vi "BLE_Thread.vi"(9 "ble queue in":refnum<queue>, 11 "controller queue out":refnum<queue>) -> ()   [LabVIEW 2020]
uses:
  BLE_Request.ctl
  BLE_Request_Command.ctl
  Controller_Request.ctl
  Controller_Request_Command.ctl
  BLE_Action.ctl
  BLE_Data_Packet.ctl
  BLE_Data.ctl
  C:/Users/Trait/Repos/BLE_BeaconSensor/BLE_ClientPC/BLELib.dll
  BLELib.dll
  BLE.lvlib
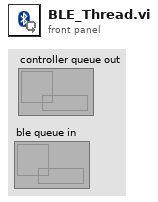
[diagram p1: front panel]
types:
  T1 = typedef "Controller_Request.ctl" = cluster{"Command":T2, "Parameter":variant}
  T2 = typedef "Controller_Request_Command.ctl" = enum16{"BLE_ScannedDevices", "BLE_ConnectionResult", "BLE_NotificationToogleResult", "BLE_NotificationData", "BLE_ConnTimeout", "BLE_CloseResult", "User_Init", "User_ScanRequest", "User_ConnectionRequest", "User_CloseRequest", "User_NotficationToggleRequest"}
  T3 = typedef "BLE_Action.ctl" = enum16{"Idle", "Notify", "Scan"}
  T4 = typedef "BLE_Data.ctl" = cluster{".NET Ref":refnum<k24>, "BLE action":T3, "Timeout":u32, "UUIDs":cluster{"TEMP":string, "ACC X":string, "ACC Y":string, "ACC Z":string}}
  T5 = typedef "BLE_Request.ctl" = cluster{"Command":T6, "Parameter":variant}
  T6 = typedef "BLE_Request_Command.ctl" = enum16{"BLE_Idle", "BLE_Init", "BLE_ScanToogle", "BLE_Connect", "BLE_NotificationToogle", "BLE_Close"}
  T7 = cluster{"TEMP":string, "ACC X":string, "ACC Y":string, "ACC Z":string}
  T8 = typedef "BLE_Data_Packet.ctl" = cluster{"Temperature":cluster{"Available":bool, "Value":sgl}, "Acceleration X":cluster{"Available":bool, "Value":i16}, "Acceleration Y":cluster{"Available":bool, "Value":i16}, "Acceleration Z":cluster{"Available":bool, "Value":i16}}
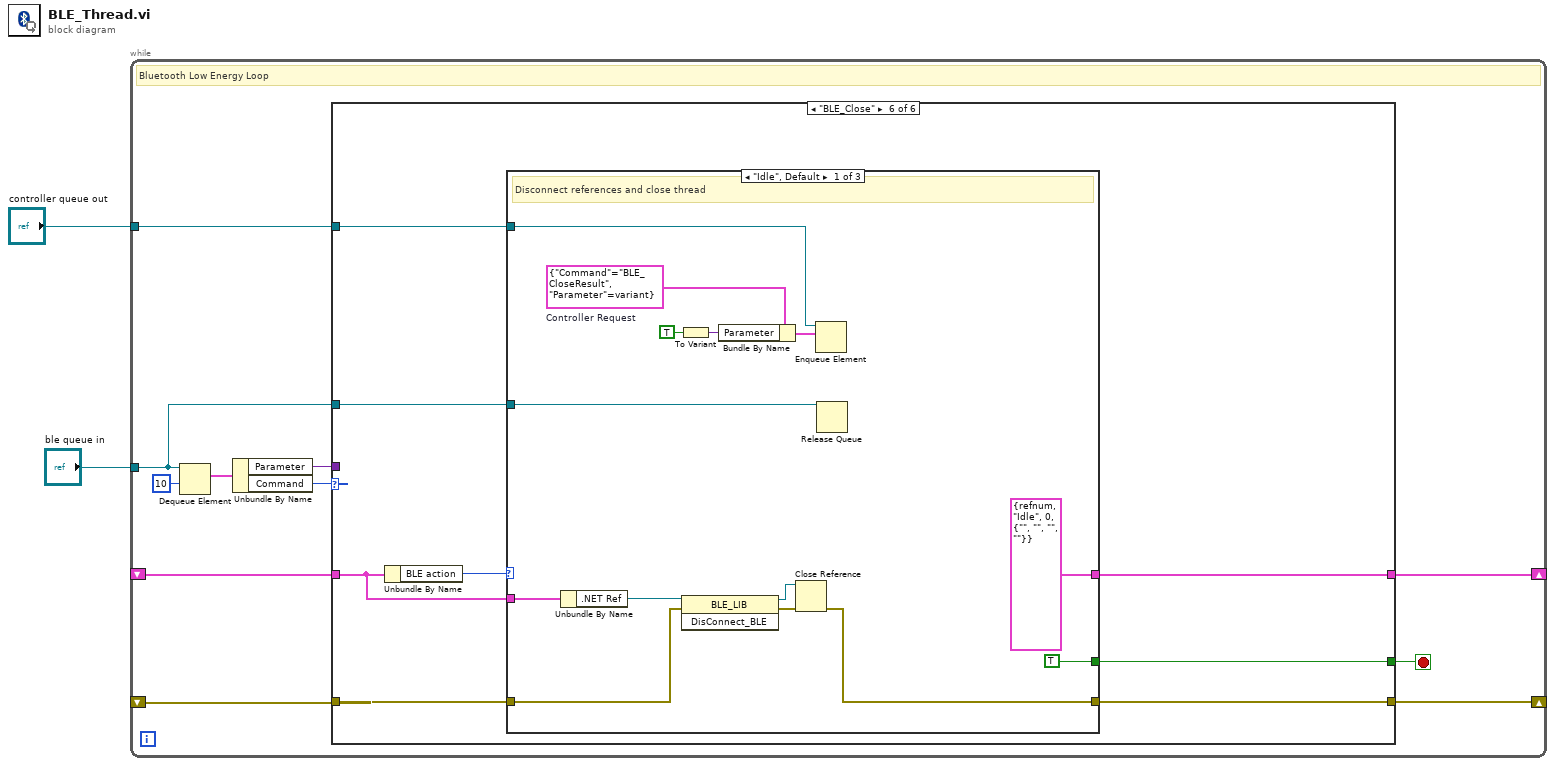
[diagram p0: block diagram]
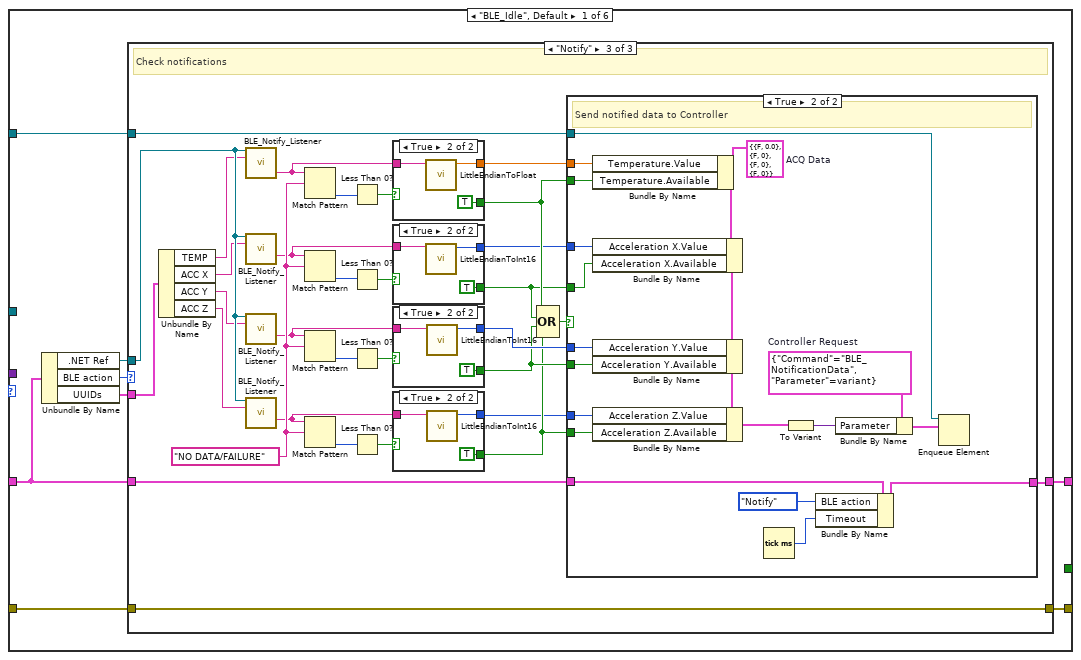
[diagram p2: hidden frame]
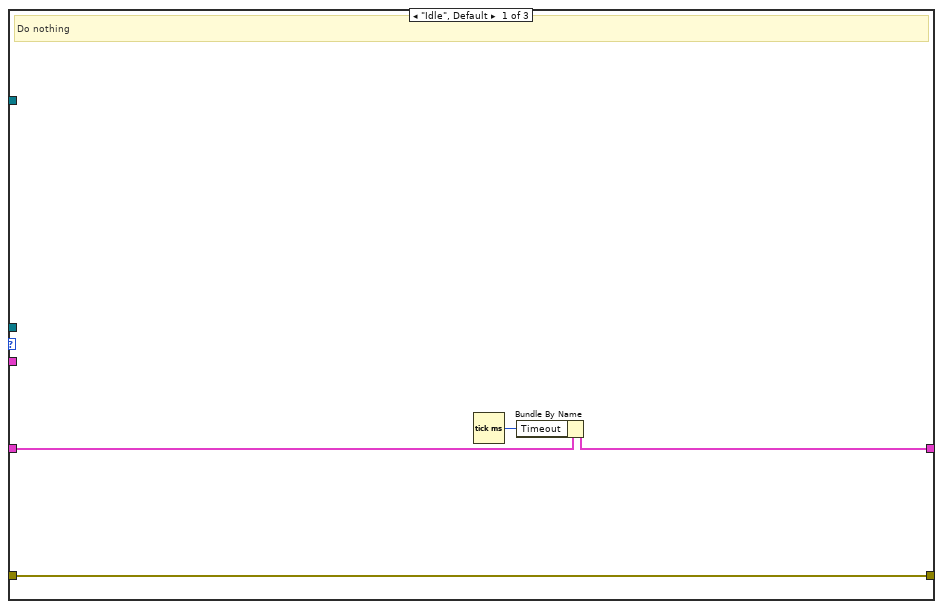
[diagram p3: hidden frame]
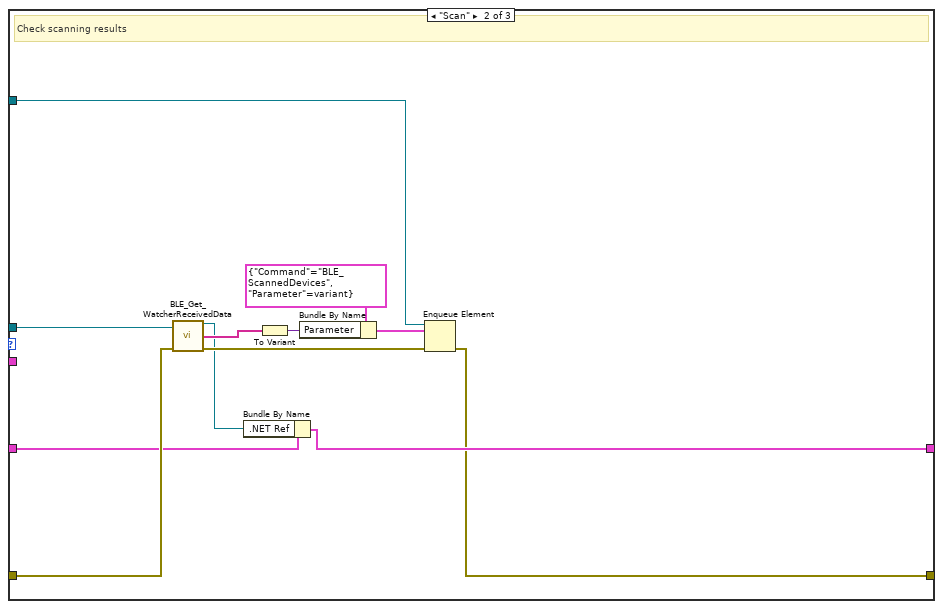
[diagram p4: hidden frame]
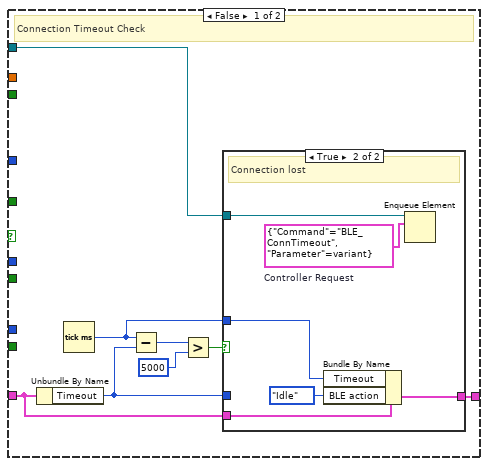
[diagram p5: hidden frame]
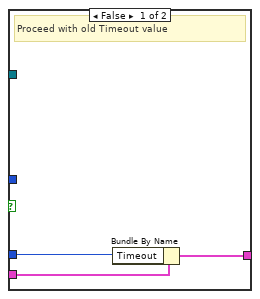
[diagram p6: hidden frame]
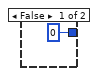
[diagram p7: hidden frame]
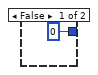
[diagram p8: hidden frame]
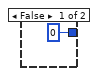
[diagram p9: hidden frame]
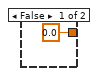
[diagram p10: hidden frame]
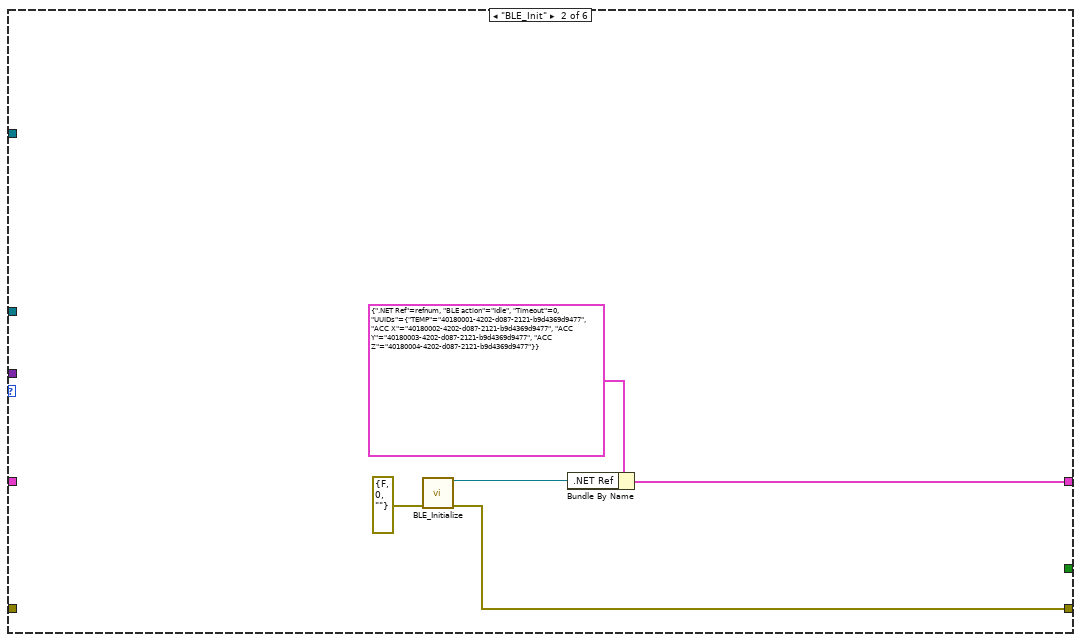
[diagram p11: hidden frame]
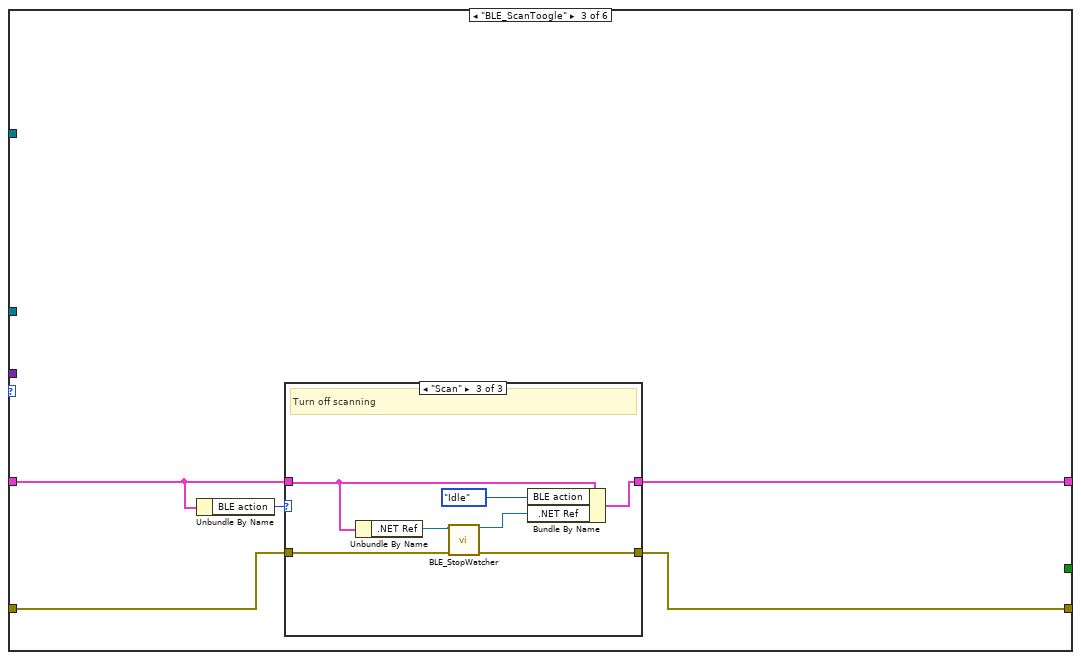
[diagram p12: hidden frame]
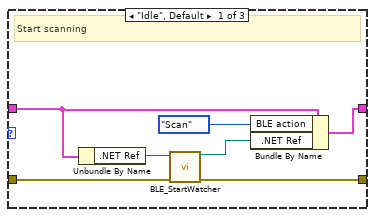
[diagram p13: hidden frame]
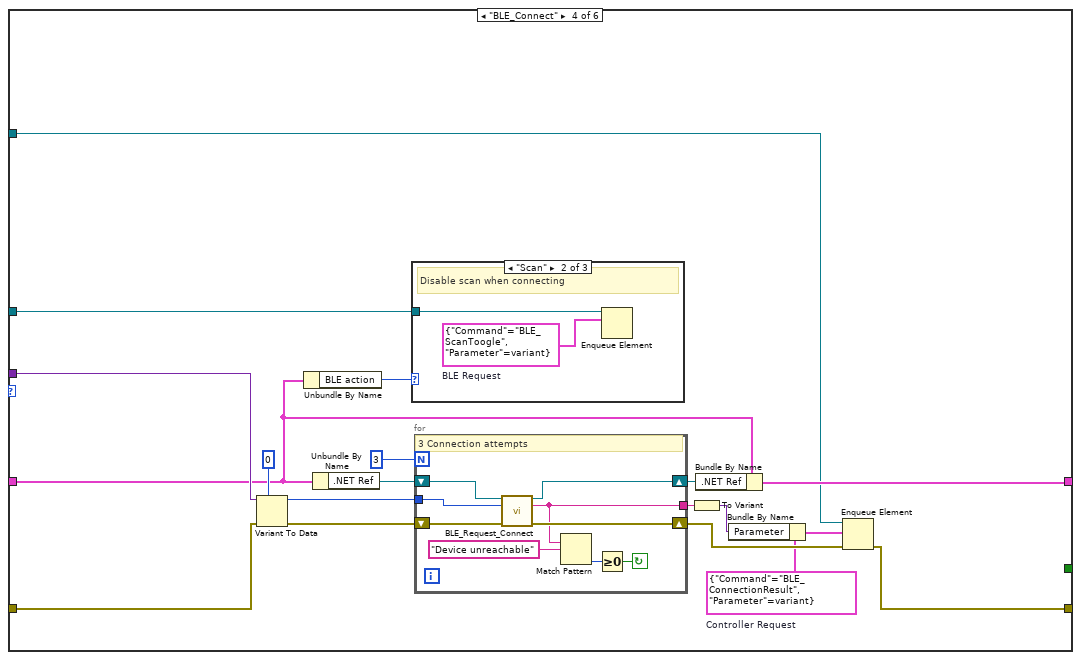
[diagram p15: hidden frame]
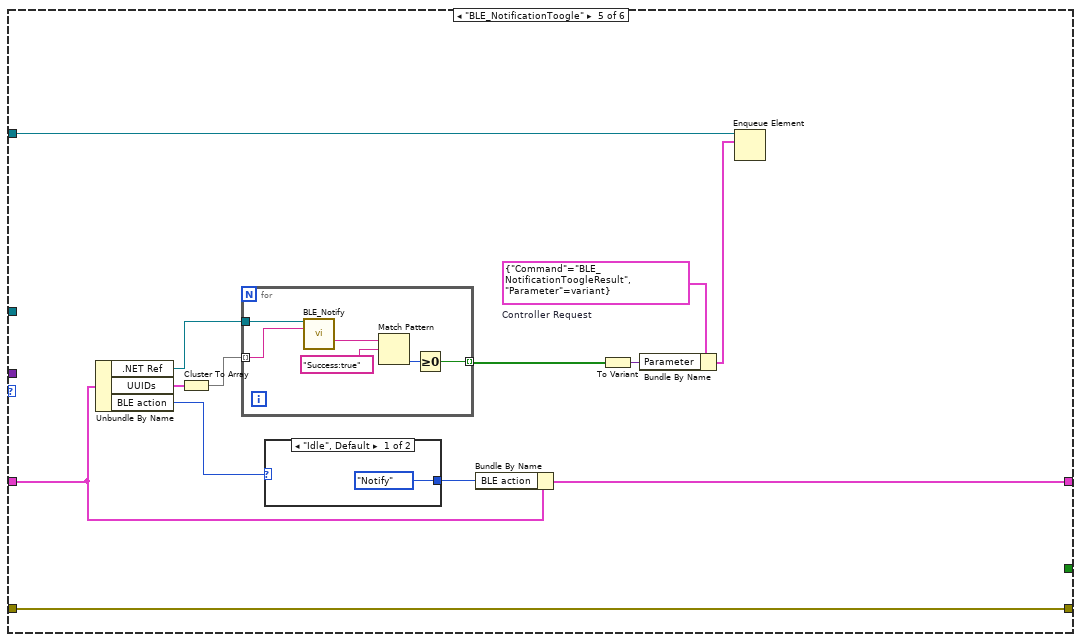
[diagram p18: hidden frame]
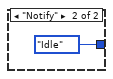
[diagram p19: hidden frame]
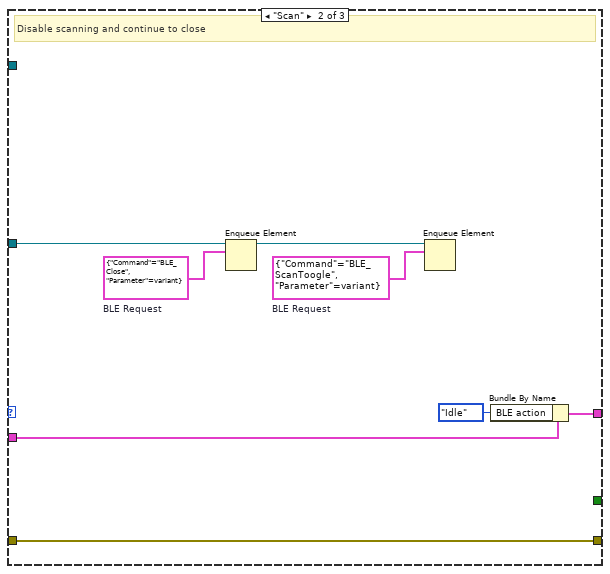
[diagram p20: hidden frame]
diagram:
  n1 = while {
    shift-right: [w4] -> _
    shift-left: _ -> [w8]
    shift-right: [w13] -> _
    shift-left: _ -> [w12]
    tunnel: "ble queue in" -> [w6]
    tunnel: "controller queue out" -> [w3]
    stop <- w5 stop-if-true
    # "Bluetooth Low Energy Loop"
    n2 = Dequeue Element(queue=w6, timeout in ms (-1)=10) -> (element=w10:T5)  [unwired: 1 in, 3 out]
    n3 = Unbundle By Name(w10) -> ("Parameter"=w7:variant, "Command"=w9:T6)
    n4 = case shown="\"BLE_Close\"" w9 {
      tunnel: w12 -> [w20 _ w130 w164 w192 w204]
      tunnel: [w16 w128 w129 w153 w192 w203] -> w13
      tunnel: [w17 w126 w133 w160 w190 w206] -> w4
      tunnel: w8 -> [w15 _ w132 w157 w191 w205]
      tunnel: w7 -> [_ _ _ w167 _ _]
      tunnel: w6 -> [_ _ _ w155 _ w207]
      tunnel: [_ _ _ _ _ w202] -> w5
      tunnel: w3 -> [w18 _ _ w152 w189 w201]
      frame "BLE_Idle", Default {
        n5 = Unbundle By Name(w15) -> (".NET Ref"=w19:refnum<k24>, "BLE action"=w21:T3, "UUIDs"=w14:T7)
        n6 = case shown="\"Notify\"" w21 {
          tunnel: w20 -> [w25 w37 w69]
          tunnel: [w25 w31 w69] -> w16
          tunnel: w15 -> [w24 w27 w39]
          tunnel: [w23 w35 w38] -> w17
          tunnel: w19 -> [_ w28 w67]
          tunnel: w18 -> [_ w29 w40]
          tunnel: w14 -> [_ _ w68]
          frame "Idle", Default {
            # "Do nothing"
            n7 = Tick Count (ms)() -> (millisecond timer value=w22:u32)
            n8 = Bundle By Name(cluster=w24, "Timeout"=w22) -> (w23:T4)
          }
          frame "Scan" {
            # "Check scanning results"
            n9 = call "BLE_Get_WatcherReceivedData.vi"(".NET Refnum in"=w28, "error in (no error)"=w37) -> (".NET Refnum out"=w26:refnum<k24>, "Bluetooth Addr"=w33:string[], "error out"=w32:errorcluster)  [unwired: 6 in, 5 out]
            n10 = Bundle By Name(cluster=w27, ".NET Ref"=w26) -> (w35:T4)
            n11 = To Variant(anything=w33) -> (Variant=w36:variant)
            n12 = Bundle By Name(cluster=T1 {"Command"=enum."BLE_ScannedDevices", "Parameter"=variant}, "Parameter"=w36) -> (w30:T1)
            n13 = Enqueue Element(queue=w29, element=w30, error in (no error)=w32) -> (error out=w31:errorcluster)  [unwired: 1 in, 2 out]
          }
          frame "Notify" {
            w55 = "NO DATA/FAILURE" ("regular expression")
            # "Check notifications"
            n14 = Unbundle By Name(w68) -> ("TEMP"=w66:string, "ACC X"=w65:string, "ACC Y"=w64:string, "ACC Z"=w63:string)
            n15 = call "BLE_Notify_Listener.vi"(".NET Refnum in"=w67, "UUID"=w66) -> ("Result"=w52:string)  [unwired: 11 in, 2 out]
            n16 = call "BLE_Notify_Listener.vi"(".NET Refnum in"=w67, "UUID"=w65) -> ("Result"=w53:string)  [unwired: 11 in, 2 out]
            n17 = call "BLE_Notify_Listener.vi"(".NET Refnum in"=w67, "UUID"=w64) -> ("Result"=w54:string)  [unwired: 11 in, 2 out]
            n18 = call "BLE_Notify_Listener.vi"(".NET Refnum in"=w67, "UUID"=w63) -> ("Result"=w51:string)  [unwired: 11 in, 2 out]
            n19 = Match Pattern(string=w52, regular expression=w55) -> (offset past match=w59:i32)  [unwired: 1 in, 3 out]
            n20 = Match Pattern(string=w53, regular expression=w55) -> (offset past match=w60:i32)  [unwired: 1 in, 3 out]
            n21 = Match Pattern(string=w54, regular expression=w55) -> (offset past match=w61:i32)  [unwired: 1 in, 3 out]
            n22 = Match Pattern(string=w51, regular expression=w55) -> (offset past match=w62:i32)  [unwired: 1 in, 3 out]
            n23 = Less Than 0?(x=w59) -> (x < 0?=w50:bool)
            n24 = Less Than 0?(x=w60) -> (x < 0?=w56:bool)
            n25 = Less Than 0?(x=w61) -> (x < 0?=w57:bool)
            n26 = Less Than 0?(x=w62) -> (x < 0?=w58:bool)
            n27 = case shown="True" w50 {
              tunnel: w52 -> [_ w123]
              tunnel: [_ TRUE] -> w49
              tunnel: [sgl 0.0 ("Float value") w121] -> w47
              frame False {
              }
              frame True {
                n28 = call "LittleEndianToFloat.vi"("Little endian float string"=w123) -> ("Float value"=w121:sgl)  [unwired: 10 in]
              }
            }
            n29 = case shown="True" w56 {
              tunnel: w53 -> [_ w119]
              tunnel: [i16 0 ("Int16 value") w118] -> w46
              tunnel: [_ TRUE] -> w45
              frame False {
              }
              frame True {
                n30 = call "LittleEndianToInt16.vi"("Little endian int string"=w119) -> ("Int16 value"=w118:i16)  [unwired: 10 in]
              }
            }
            n31 = case shown="True" w57 {
              tunnel: w54 -> [_ w115]
              tunnel: [i16 0 ("Int16 value") w114] -> w44
              tunnel: [_ TRUE] -> w43
              frame False {
              }
              frame True {
                n32 = call "LittleEndianToInt16.vi"("Little endian int string"=w115) -> ("Int16 value"=w114:i16)  [unwired: 10 in]
              }
            }
            n33 = case shown="True" w58 {
              tunnel: w51 -> [_ w111]
              tunnel: [i16 0 ("Int16 value") w110] -> w41
              tunnel: [_ TRUE] -> w42
              frame False {
              }
              frame True {
                n34 = call "LittleEndianToInt16.vi"("Little endian int string"=w111) -> ("Int16 value"=w110:i16)  [unwired: 10 in]
              }
            }
            n35 = Compound Arithmetic op=OR(w49, w45, w43, w42) -> (w48:bool)
            n36 = case shown="True" w48 {
              tunnel: w49 -> [_ w106]
              tunnel: w47 -> [_ w105]
              tunnel: w46 -> [_ w103]
              tunnel: w45 -> [_ w102]
              tunnel: w44 -> [_ w101]
              tunnel: w43 -> [_ w100]
              tunnel: w42 -> [_ w98]
              tunnel: w41 -> [_ w97]
              tunnel: w40 -> [w73 w95]
              tunnel: w39 -> [w72 w93]
              tunnel: [w71 w89] -> w38
              frame False {
                # "Connection Timeout Check"
                n37 = Unbundle By Name(w72) -> ("Timeout"=w77:u32)
                n38 = Tick Count (ms)() -> (millisecond timer value=w70:u32)
                n39 = Subtract(x=w70, y=w77) -> (x-y=w75:u32)
                n40 = Greater?(x=w75, y=u32 5000) -> (0:w76:bool)
                n41 = case shown="True" w76 {
                  tunnel: w77 -> [w78 _]
                  tunnel: w73 -> [_ w85]
                  tunnel: w72 -> [w80 w84]
                  tunnel: [w79 w83] -> w71
                  tunnel: w70 -> [_ w81]
                  frame False {
                    # "Proceed with old Timeout value"
                    n42 = Bundle By Name(cluster=w80, "Timeout"=w78) -> (w79:T4)
                  }
                  frame True {
                    w86 = T1 {"Command"=enum."BLE_ConnTimeout", "Parameter"=variant}  # Controller Request
                    # "Connection lost"
                    n43 = Bundle By Name(cluster=w84, "Timeout"=w81, "BLE action"=BLE_Action."Idle") -> (w83:T4)
                    n44 = Enqueue Element(queue=w85, element=w86) -> ()  [unwired: 2 in, 3 out]
                  }
                }
              }
              frame True {
                w92 = T1 {"Command"=enum."BLE_NotificationData", "Parameter"=variant}  # Controller Request
                w107 = T8 {"Temperature"={"Available"=FALSE, "Value"=0.0}, "Acceleration X"={"Available"=FALSE, "Value"=0}, "Acceleration Y"={"Available"=FALSE, "Value"=0}, "Acceleration Z"={"Available"=FALSE, "Value"=0}}  # ACQ Data
                # "Send notified data to Controller"
                n45 = Bundle By Name(cluster=w107, "Temperature.Value"=w105, "Temperature.Available"=w106) -> (w104:T8)
                n46 = Bundle By Name(cluster=w104, "Acceleration X.Value"=w103, "Acceleration X.Available"=w102) -> (w99:T8)
                n47 = Bundle By Name(cluster=w99, "Acceleration Y.Value"=w101, "Acceleration Y.Available"=w100) -> (w96:T8)
                n48 = Bundle By Name(cluster=w96, "Acceleration Z.Value"=w97, "Acceleration Z.Available"=w98) -> (w94:T8)
                n49 = Tick Count (ms)() -> (millisecond timer value=w87:u32)
                n50 = To Variant(anything=w94) -> (Variant=w90:variant)
                n51 = Bundle By Name(cluster=w93, "BLE action"=BLE_Action."Notify", "Timeout"=w87) -> (w89:T4)
                n52 = Bundle By Name(cluster=w92, "Parameter"=w90) -> (w91:T1)
                n53 = Enqueue Element(queue=w95, element=w91) -> ()  [unwired: 2 in, 3 out]
              }
            }
          }
        }
      }
      frame "BLE_Init" {
        n54 = call "BLE_Initialize.vi"("error in (no error)"=errorcluster {"status"=FALSE, "code"=0, "source"=""} ("error constant")) -> (".NET Refnum out"=w127:refnum<k24>, "error out"=w128:errorcluster)  [unwired: 13 in]
        n55 = Bundle By Name(cluster=T4 {".NET Ref"=refnum, "BLE action"=enum."Idle", "Timeout"=0, "UUIDs"={"TEMP"="40180001-4202-d087-2121-b9d4369d9477", "ACC X"="40180002-4202-d087-2121-b9d4369d9477", "ACC Y"="40180003-4202-d087-2121-b9d4369d9477", "ACC Z"="40180004-4202-d087-2121-b9d4369d9477"}}, ".NET Ref"=w127) -> (w126:T4)
      }
      frame "BLE_ScanToogle" {
        n56 = Unbundle By Name(w132) -> ("BLE action"=w131:T3)
        n57 = case shown="\"Scan\"" w131 {
          tunnel: w132 -> [w139 w142 w148]
          tunnel: [w135 w142 w147] -> w133
          tunnel: w130 -> [w134 w141 w144]
          tunnel: [w136 w141 w143] -> w129
          frame "Idle", Default {
            # "Start scanning"
            n58 = Unbundle By Name(w139) -> (".NET Ref"=w138:refnum<k24>)
            n59 = call "BLE_StartWatcher.vi"(".NET Refnum in"=w138, "error in (no error)"=w134) -> (".NET Refnum out"=w137:refnum<k24>, "error out"=w136:errorcluster)  [unwired: 11 in, 1 out]
            n60 = Bundle By Name(cluster=w139, "BLE action"=BLE_Action."Scan" ("Idle action"), ".NET Ref"=w137) -> (w135:T4)
          }
          frame "Notify" {
            # "Scanning not available when notifications on"
          }
          frame "Scan" {
            # "Turn off scanning"
            n61 = Unbundle By Name(w148) -> (".NET Ref"=w149:refnum<k24>)
            n62 = call "BLE_StopWatcher.vi"(".NET Refnum in"=w149, "error in (no error)"=w144) -> (".NET Refnum out"=w145:refnum<k24>, "error out"=w143:errorcluster)  [unwired: 11 in, 1 out]
            n63 = Bundle By Name(cluster=w148, "BLE action"=BLE_Action."Idle" ("Idle action"), ".NET Ref"=w145) -> (w147:T4)
          }
        }
      }
      frame "BLE_Connect" {
        w151 = T1 {"Command"=enum."BLE_ConnectionResult", "Parameter"=variant}  # Controller Request
        n64 = Variant To Data(error in=w164, type=u64 0, Variant=w167) -> (data=w165:u64, error out=w163:errorcluster)
        n65 = Unbundle By Name(w157) -> ("BLE action"=w156:T3)
        n66 = Unbundle By Name(w157) -> (".NET Ref"=w168:refnum<k24>)
        n67 = case shown="\"Scan\"" w156 {
          tunnel: w155 -> [_ w170 _]
          frame "Idle", Default {
          }
          frame "Scan" {
            w169 = T5 {"Command"=enum."BLE_ScanToogle", "Parameter"=variant}  # BLE Request
            # "Disable scan when connecting"
            n68 = Enqueue Element(queue=w170, element=w169) -> ()  [unwired: 2 in, 3 out]
          }
          frame "Notify" {
          }
        }
        n69 = for {
          N: 3 -> [_]
          tunnel: w165 -> [w178]
          shift-right: [w174] -> w161
          shift-left: w168 -> [w179]
          shift-right: [w172] -> w154
          shift-left: w163 -> [w177]
          tunnel: [w171] -> w159
          stop <- w173 continue-if-true
          # "3 Connection attempts"
          n70 = call "BLE_Request_Connect.vi"(".NET Refnum in"=w179, "BluetoothAddress"=w178, "error in (no error)"=w177) -> (".NET Refnum out"=w174:refnum<k24>, "ConnectBLE"=w171:string, "error out"=w172:errorcluster)  [unwired: 10 in]
          n71 = Match Pattern(string=w171, regular expression="Device unreachable") -> (offset past match=w176:i32)  [unwired: 1 in, 3 out]
          n72 = Greater Or Equal To 0?(x=w176) -> (x >= 0?=w173:bool)
        }
        n73 = To Variant(anything=w159) -> (Variant=w158:variant)
        n74 = Bundle By Name(cluster=w157, ".NET Ref"=w161) -> (w160:T4)
        n75 = Bundle By Name(cluster=w151, "Parameter"=w158) -> (w150:T1)
        n76 = Enqueue Element(queue=w152, element=w150, error in (no error)=w154) -> (error out=w153:errorcluster)  [unwired: 1 in, 2 out]
      }
      frame "BLE_NotificationToogle" {
        w188 = T1 {"Command"=enum."BLE_NotificationToogleResult", "Parameter"=variant}  # Controller Request
        n77 = Unbundle By Name(w191) -> (".NET Ref"=w184:refnum<k24>, "UUIDs"=w182:T7, "BLE action"=w181:T3)
        n78 = Cluster To Array(cluster=w182) -> (array=w183:string[])
        n79 = for {
          tunnel: w184 -> [w195]
          tunnel: w183 -> [w194] mode=indexing
          tunnel: [w193] -> w180 mode=indexing
          n80 = call "BLE_Notify.vi"(".NET Refnum in"=w195, "UUID"=w194) -> ("Result"=w196:string)  [unwired: 11 in, 2 out]
          n81 = Match Pattern(string=w196, regular expression="Success:true") -> (offset past match=w198:i32)  [unwired: 1 in, 3 out]
          n82 = Greater Or Equal To 0?(x=w198) -> (x >= 0?=w193:bool)
        }
        n83 = case shown="\"Idle\", Default" w181 {
          tunnel: [BLE_Action."Notify" ("BLE action") BLE_Action."Idle" ("BLE action")] -> w185
          frame "Idle", Default {
          }
          frame "Notify" {
          }
        }
        n84 = Bundle By Name(cluster=w191, "BLE action"=w185) -> (w190:T4)
        n85 = To Variant(anything=w180) -> (Variant=w186:variant)
        n86 = Bundle By Name(cluster=w188, "Parameter"=w186) -> (w187:T1)
        n87 = Enqueue Element(queue=w189, element=w187) -> ()  [unwired: 2 in, 3 out]
      }
      frame "BLE_Close" {
        n88 = Unbundle By Name(w205) -> ("BLE action"=w208:T3)
        n89 = case shown="\"Idle\", Default" w208 {
          tunnel: w207 -> [w209 w230 w234]
          tunnel: [T4 {".NET Ref"=refnum, "BLE action"=enum."Idle", "Timeout"=0, "UUIDs"={"TEMP"="", "ACC X"="", "ACC Y"="", "ACC Z"=""}} w228 w232] -> w206
          tunnel: w205 -> [w222 w227 w233]
          tunnel: w204 -> [w216 w226 w231]
          tunnel: [w215 w226 w231] -> w203
          tunnel: [TRUE _ _] -> w202
          tunnel: w201 -> [w214 _ _]
          frame "Idle", Default {
            w213 = T1 {"Command"=enum."BLE_CloseResult", "Parameter"=variant}  # Controller Request
            # "Disconnect references and close thread"
            n90 = Unbundle By Name(w222) -> (".NET Ref"=w219:refnum<k24>)
            n91 = To Variant(anything=TRUE) -> (Variant=w211:variant)
            n92 = invoke class="BLE_LIB" method="DisConnect_BLE"(reference=w219, error in=w216) -> (reference out=w221:refnum<k24>, error out=w220:errorcluster)  [unwired: 1 in, 1 out]
            n93 = Bundle By Name(cluster=w213, "Parameter"=w211) -> (w212:T1)
            n94 = Close Reference(reference=w221, error in (no error)=w220) -> (error out=w215:errorcluster)
            n95 = Enqueue Element(queue=w214, element=w212) -> ()  [unwired: 2 in, 3 out]
            n96 = Release Queue(queue=w209) -> ()  [unwired: 2 in, 3 out]
          }
          frame "Scan" {
            w223 = T5 {"Command"=enum."BLE_Close", "Parameter"=variant}  # BLE Request
            w224 = T5 {"Command"=enum."BLE_ScanToogle", "Parameter"=variant}  # BLE Request
            # "Disable scanning and continue to close"
            n97 = Enqueue Element(queue=w230, element=w223) -> (queue out=w229:refnum<queue>)  [unwired: 2 in, 2 out]
            n98 = Enqueue Element(queue=w229, element=w224) -> ()  [unwired: 2 in, 3 out]
            n99 = Bundle By Name(cluster=w227, "BLE action"=BLE_Action."Idle") -> (w228:T4)
          }
          frame "Notify" {
            w237 = T5 {"Command"=enum."BLE_Close", "Parameter"=variant}  # BLE Request
            w236 = T5 {"Command"=enum."BLE_NotificationToogle", "Parameter"=variant}  # BLE Request
            # "Disable notifications and continue to close"
            n100 = Enqueue Element(queue=w234, element=w237) -> (queue out=w238:refnum<queue>)  [unwired: 2 in, 2 out]
            n101 = Enqueue Element(queue=w238, element=w236) -> ()  [unwired: 2 in, 3 out]
            n102 = Bundle By Name(cluster=w233, "BLE action"=BLE_Action."Idle") -> (w232:T4)
          }
        }
      }
    }
  }
